vi "projectSineWave.vi"(10 "colors":u32[](array[numeric]), 11 "8-bit pixmap":u8[][](array[numeric])) -> (1 "projSize":i32[](array[numeric]), 3 "new picture":picture)   [LabVIEW 2017]
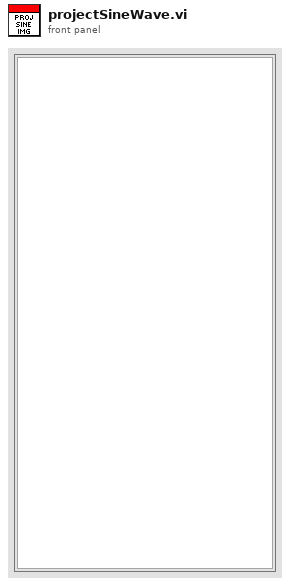
[diagram p1: front panel]
types:
  T1 = typedef "imagedata.ctl" = cluster{"image type":i32, "image depth":i32, "image":u8[], "mask":u8[], "colors":u32[], "Rectangle":cluster{"left":i16, "top":i16, "right":i16, "bottom":i16}}
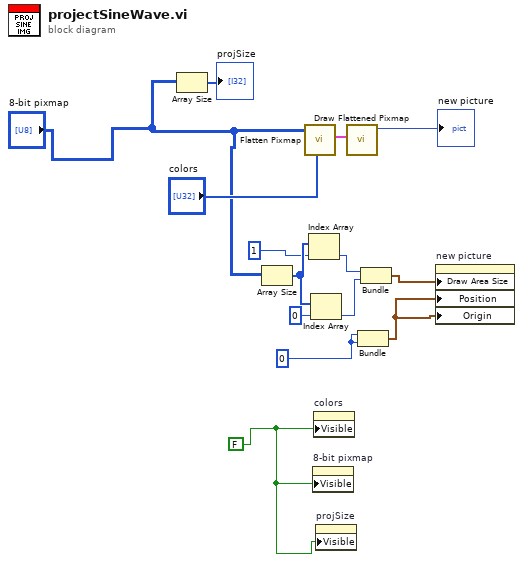
[diagram p0: block diagram]
diagram:
  w3 = FALSE
  w1 = 0
  n1 = Array Size(array="8-bit pixmap") -> (size(s)=→"projSize":i32[])
  n2 = Array Size(array="8-bit pixmap") -> (size(s)=w10:i32[])
  n3 = call <vilib>:"Flatten Pixmap.vi"("colors"="colors", "8-bit pixmap"="8-bit pixmap") -> ("image data"=w13:T1)  [unwired: 9 in]
  n4 = Index Array(array=w10, index=1) -> (element=w7:i32)
  n5 = Index Array(array=w10, index=0) -> (element=w6:i32)
  n6 = property on="8-bit pixmap" class="Arr (strict)"("Visible"=w3) -> ()  [unwired: 2 in, 2 out]
  n7 = property on="colors" class="Arr (strict)"("Visible"=w3) -> ()  [unwired: 2 in, 2 out]
  n8 = property on="projSize" class="Arr (strict)"("Visible"=w3) -> ()  [unwired: 2 in, 2 out]
  n9 = call <vilib>:"Draw Flattened Pixmap.vi"("image data"=w13) -> ("new picture"=→"new picture":picture)  [unwired: 8 in]
  n10 = Bundle(w1, w1) -> (w11:cluster{i32, i32})  [unwired: 1 in]
  n11 = Bundle(w7, w6) -> (w5:cluster{i32, i32})  [unwired: 1 in]
  n12 = property on="new picture" class="Pict"("Draw Area Size"=w5, "Position"=w11, "Origin"=w11) -> ()  [unwired: 2 in, 2 out]
